vi "Open and Config Port.vi"(8 "error in (no error)":errorcluster, 11 "Serial Client in":refnum<class "Serial Client.lvclass">) -> (0 "error out":errorcluster, 2 "VISA resource name out":refnum<visa-resource-name>, 3 "Serial Client":refnum<class "Serial Client.lvclass">)   [LabVIEW 2020, in "Stream-Serial.lvlib" / "Serial Client.lvclass"]
uses:
  Serial Client.lvclass
  Serial Client.lvclass/Serial Client.ctl
  <vilib>/IlluminatedG/lv-stream/URI/URI.lvclass
  <vilib>/IlluminatedG/lv-stream/Endpoint/Endpoint.lvclass
  <vilib>/Instr/_visa.llb/VISA Configure Serial Port (Instr).vi
  C:/Program Files (x86)/National Instruments/LabVIEW 2020/vi.lib/IlluminatedG/lv-stream/Connection/Connection.lvclass
  C:/Program Files (x86)/National Instruments/LabVIEW 2020/vi.lib/IlluminatedG/lv-stream/Endpoint/Endpoint.lvclass
  C:/dev/lv 2020/lv-stream-serial/Stream-Serial/Serial Client/Serial Client.lvclass
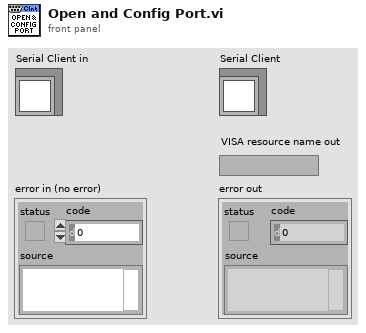
[diagram p1: front panel]
types:
  T1 = typedef "Stream-Serial.lvlib/Serial Client.lvclass/Port Config.ctl" = cluster{"Baud (115200)":u32, "Data Bits (8)":u8, "Stop Bits (1)":T2, "Flow Control":T3, "Use LineTerm?":bool, "LineTerm (\\n)":string, "Timeout ms (10000)":i32, "Parity (None)":T4}
  T2 = typedef "Stream-Serial.lvlib/Serial Client.lvclass/Stop Bits.ctl" = u16
  T3 = typedef "Stream-Serial.lvlib/Serial Client.lvclass/Flow Control.ctl" = u16
  T4 = typedef "Stream-Serial.lvlib/Serial Client.lvclass/Parity.ctl" = enum16{"None", "Odd", "Even", "Mark", "Space"}
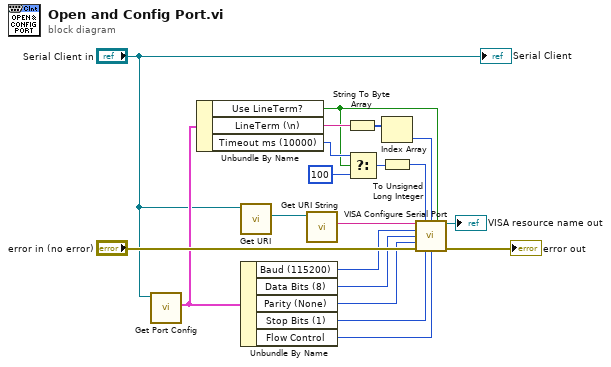
[diagram p0: block diagram]
diagram:
  n1 = call "Get Port Config.vi"("Serial Client in"="Serial Client in") -> ("Port Config"=w10:T1)  [unwired: 8 in, 2 out]
  n2 = Unbundle By Name(w10) -> ("Use LineTerm?"=w1:bool, "LineTerm (\\n)"=w9:string, "Timeout ms (10000)"=w6:i32)
  n3 = call <vilib>:"Get URI.vi"("Endpoint in"="Serial Client in") -> ("URI"=w14:refnum<class "URI.lvclass">)  [unwired: 8 in, 2 out]
  n4 = Unbundle By Name(w10) -> ("Baud (115200)"=w19:u32, "Data Bits (8)"=w18:u8, "Parity (None)"=w17:T4, "Stop Bits (1)"=w16:T2, "Flow Control"=w15:T3)
  n5 = call <vilib>:"Get URI String.vi"("URI in"=w14) -> ("URI String"=w13:string)  [unwired: 8 in, 2 out]
  n6 = String To Byte Array(string=w9) -> (unsigned byte array=w8:u8[])
  n7 = Select(t=w6, s=w1, f=100) -> (s? t:f=w4:i32)
  n8 = Index Array(array=w8) -> (element=w7:u8)  [unwired: 1 in]
  n9 = To Unsigned Long Integer(number=w4) -> (unsigned 32bit integer=w3:u32)
  n10 = call-poly "VISA Configure Serial Port"("VISA resource name"=w13, "timeout (10sec)"=w3, "termination char\n(0xA = '\\n' = LF)"=w7, "Enable Termination\nChar (T)"=w1, "baud rate (9600)"=w19, "data bits (8)"=w18, "parity (0:none)"=w17, "error in (no error)"="error in (no error)", "stop bits (10: 1 bit)"=w16, "flow control (0:none)"=w15) -> ("VISA resource name out"=→"VISA resource name out":refnum<visa-resource-name>, "error out"=→"error out":errorcluster)  [unwired: 4 in]
  "Serial Client" <- "Serial Client in"
